vi "MatchEmbedByGUID.vi"(8 "error in (no error)":errorcluster, 10 "GUID":string, 11 "SMO.UI.MAUI in":refnum<class "MAUI.lvclass">) -> (0 "error out":errorcluster, 1 "Index":i32, 2 "Value":refnum<class "Embedded UI.lvclass">, 3 "SMO.UI.MAUI out":refnum<class "MAUI.lvclass">, 4 "Found?":bool)   [LabVIEW 2019, in "MAUI.lvclass"]
uses:
  MAUI.lvclass
  <vilib>/JKI/JKI SMO/SMO/SMO.lvclass
  <userlib>/LevyLab/Embedded UI/Embedded UI/Embedded UI.lvclass
  C:/Program Files (x86)/National Instruments/LabVIEW 2019/vi.lib/JKI/JKI SMO/SMO/SMO.lvclass
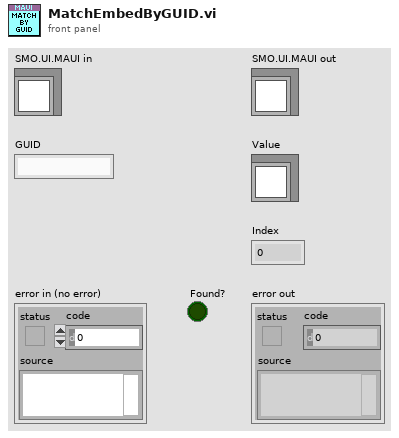
[diagram p1: front panel]
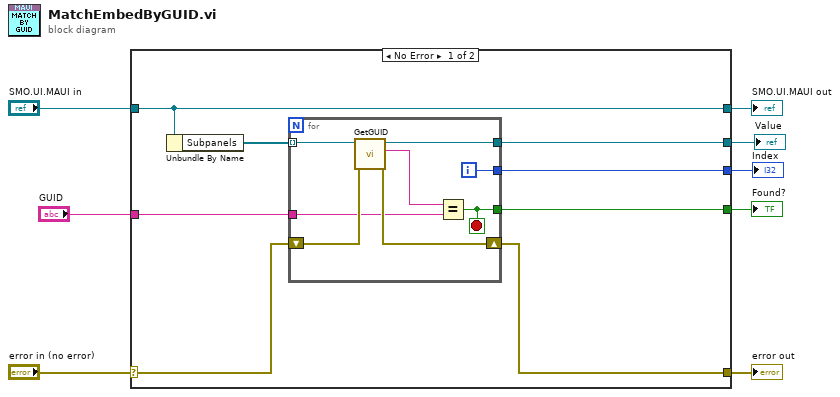
[diagram p0: block diagram]
diagram:
  n1 = case shown="No Error" "error in (no error)" {
    selector: "error in (no error)" -> [w16 w26]
    tunnel: [w15 w26] -> w7
    tunnel: [w14 w25] -> w5
    tunnel: "SMO.UI.MAUI in" -> [w14 w25]
    tunnel: "GUID" -> [w12 _]
    tunnel: [w11 _] -> w3
    tunnel: [w10 _] -> w2
    tunnel: [w9 _] -> w1
    frame No Error {
      n2 = Unbundle By Name(w14) -> ("Subpanels"=w13:refnum<class "Embedded UI.lvclass">[])
      n3 = for {
        tunnel: w13 -> [w22] mode=indexing
        tunnel: w12 -> [w20]
        shift-right: [w23] -> w15
        shift-left: w16 -> [w24]
        tunnel: [w19] -> w10
        tunnel: [w18] -> w11
        tunnel: [w17] -> w9
        i -> [w19]
        stop <- w17 stop-if-true
        n4 = call <vilib>:"GetGUID.vi"("error in (no error)"=w24, "SMO"=w22) -> ("error out"=w23:errorcluster, "GUID"=w21:string, "SMO out"=w18:refnum<class "Embedded UI.lvclass">)  [unwired: 7 in]
        n5 = Equal?(x=w21, y=w20) -> (x = y?=w17:bool)
      }
    }
    frame Error {
    }
  }
  "error out" <- w7
  "SMO.UI.MAUI out" <- w5
  "Value" <- w3
  "Index" <- w2
  "Found?" <- w1
